vi "brc_daq_get_parameters.vi"(5 "error in (no error)":errorcluster, 6 "mHandle":i32) -> (14 "sample_rate":dbl, 15 "coupling_mode":i32, 16 "current":dbl, 19 "error out":errorcluster)   [LabVIEW 2019, in "BRC-DAQ.lvlib"]
uses:
  BRC-DAQ.lvlib
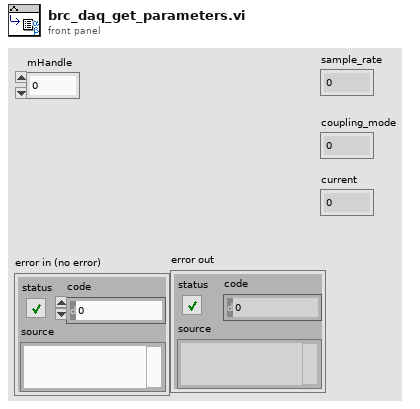
[diagram p1: front panel]
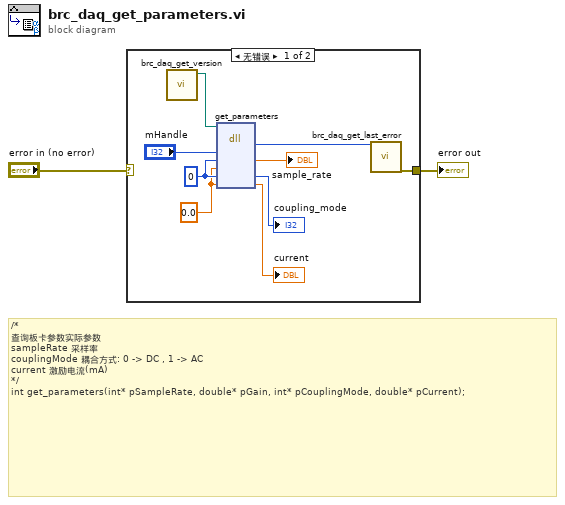
[diagram p0: block diagram]
diagram:
  # "/*\n查询板卡参数实际参数\nsampleRate 采样率\ncouplingMode 耦合方式: 0 -> DC , 1 -> AC\ncurrent 激励电流(mA)\n*/\nint get_parameters(int* pSampleRate, double* pGain, int* pCouplingMode, double* pCurrent);"
  n1 = case shown="无错误" "error in (no error)" {
    selector: "error in (no error)" -> [_ w12]
    tunnel: [w7 w12] -> w2
    frame No Error {
      w6 = 0 ("sampleRate")
      w5 = 0.0 ("pGain")
      n2 = call "brc_daq_get_version.vi"() -> ("dll path"=w3:path)  [unwired: 11 in]
      n3 = dll-call lib="E:/01 BRC project/04BRC-daq/04 Drive/DAQ-x64/DLL/brc_daq_sdk.dll" fn="get_parameters"(path in=w3, "mHandle"="mHandle", "sampleRate"=w6, "Gain"=w5, "couplingMode"=w6, "current"=w5) -> ("return type"=w8:i32, "sampleRate"=→"sample_rate":dbl, "couplingMode"=→"coupling_mode":i32, "current"=→"current":dbl)  [unwired: 4 in, 2 out]
      n4 = call "brc_daq_get_last_error.vi"("return_value"=w8) -> ("error out"=w7:errorcluster)  [unwired: 18 in]
    }
    frame Error {
    }
  }
  "error out" <- w2
